vi "_[error50001]Can't Found Value.vi"(8 "error in (no error)":errorcluster, 10 "db name":string, 11 "value name":string) -> (0 "error out":errorcluster)   [LabVIEW 2017, in "TagDB.lvlib"]
uses:
  TagDB.lvlib
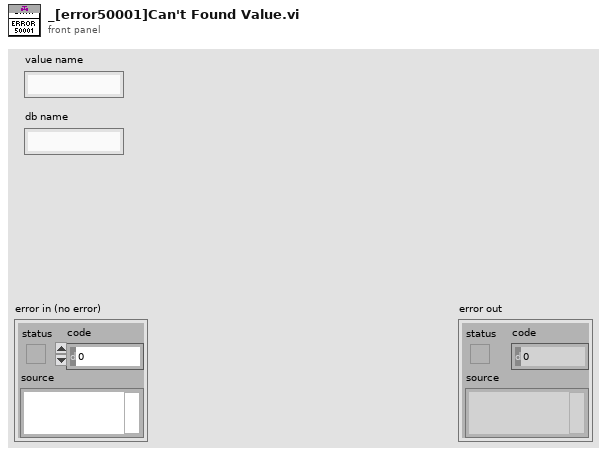
[diagram p1: front panel]
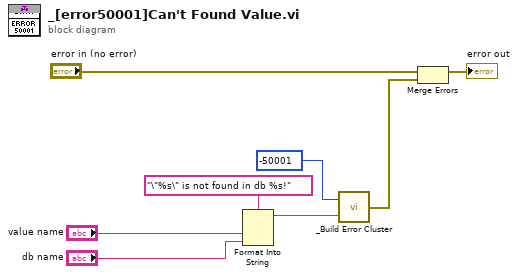
[diagram p0: block diagram]
diagram:
  n1 = Format Into String(format string="\"%s\" is not found in db %s!" ("source"), "value name", "db name") -> (resulting string=w3:string)  [unwired: 2 in, 1 out]
  n2 = call "_Build Error Cluster.vi"("String to Prepend to source (\"\")"=w3, "code"=-50001) -> ("error out"=w2:errorcluster)
  n3 = Merge Errors("error in (no error)", w2) -> (→"error out":errorcluster)
